vi "Sync Internal Phase.vi"(8 "error in (no error)":errorcluster, 11 "VISA resource name":refnum<visa-resource-name>) -> (0 "error out":errorcluster, 3 "VISA resource name out":refnum<visa-resource-name>)   [LabVIEW 2026, in "Agilent 3352X Series.lvlib"]
doc: "Simultaneously resets all phase generators in the instrument to establish a common, internal phase zero reference point. \nFor example. You can synchronize the phase between the primary signal and the sum signal by this VI\n\n<b>Note</b>:\nThis VI breaks the phase relation with another instrument, because it resets the phase generators."
uses:
  Agilent 3352X Series.lvlib
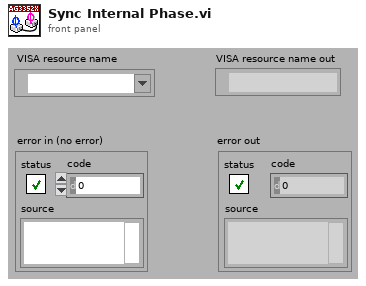
[diagram p1: front panel]
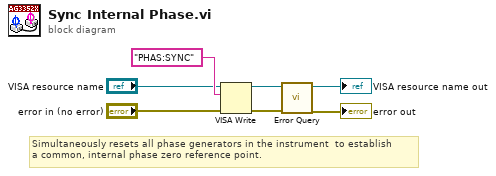
[diagram p0: block diagram]
diagram:
  # "Simultaneously resets all phase generators in the instrument  to establish \na common, internal phase zero reference point."
  n1 = VISA Write(VISA resource name="VISA resource name", write buffer="PHAS:SYNC", error in (no error)="error in (no error)") -> (VISA resource name out=w4:refnum<visa-resource-name>, error out=w3:errorcluster)  [unwired: 1 out]
  n2 = call "Error Query.vi"("error in (no error)"=w3, "VISA resource name"=w4) -> ("error out"=→"error out":errorcluster, "VISA resource name out"=→"VISA resource name out":refnum<visa-resource-name>)  [unwired: 8 out]
